vi "Evaluate.vi"(8 "error in (no error)":errorcluster, 10 "Point":dbl[](array[numeric]), 11 "TestObjetive in":refnum<class "TestObjetive.lvclass">) -> (0 "error out":errorcluster, 2 "evaluation":dbl, 3 "TestObjetive out":refnum<class "TestObjetive.lvclass">)   [LabVIEW 2023, in "TestObjetive.lvclass"]
uses:
  TestObjetive.lvclass
  TestObjetive.lvclass/TestObjetive.ctl
  Team_class/OffensivePlay.ctl
  Utilities_class/Utilities.lvclass
panel:
  in  "nearGoal":dbl=1.0 format="%#_13g"
  in  "enemyInSquare":dbl=1.0 format="%#_13g"
  in  "dangerEnemy":dbl=1.0 format="%#_13g"
  in  "factorPass":dbl=1.0 format="%#_13g"
  in  "bestY":dbl=1.0 format="%#_13g"
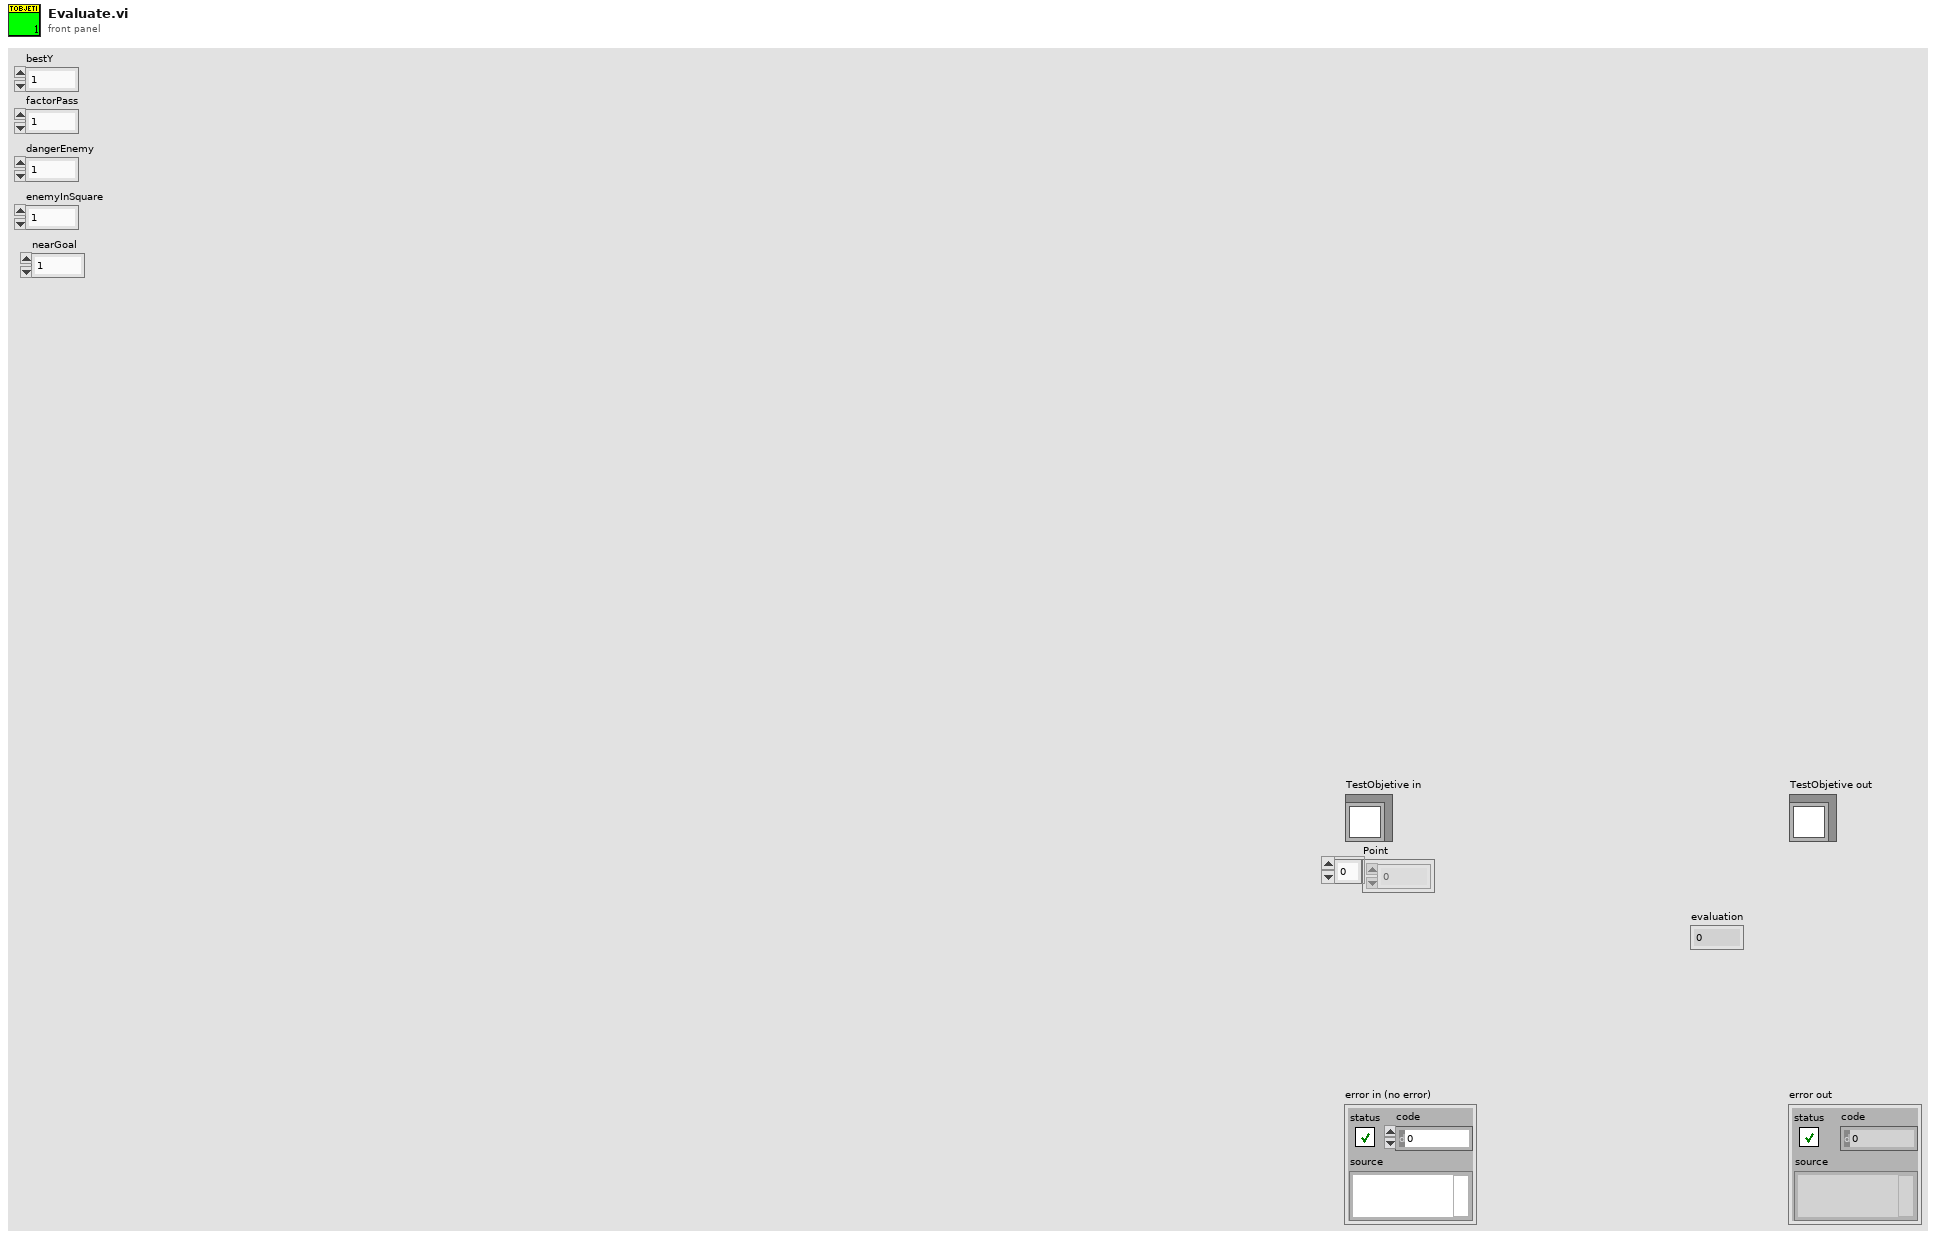
[diagram p1: front panel]
types:
  T1 = typedef "OffensivePlay.ctl" = enum16{"5RobotsPassGamePlay", "5PreparePassGame", "5RobotsKeeperGame", "KeeperPassToStriker", "5RobotsNormalGamePlay", "PrepareKeeperPass", "ACBPass", "ABCPass", "PrepareTriplePass", "TableWithStriker", "TableWith2ndStrikerPlay", "PrepareDoublePass", "PrepareRollToPass", "SimplePass", "PreparePass", "PassToStriker", "BallOutOfField", "PassTo2ndStriker", "StopOffensive", "Prepare Penalty Enemy", "EnemyPossessionAtEnemyField", "EnemyPossesionAtOurField", "TestPlay", "PreparePenaltyAlly", "KickPenaltyAlly", "PrepareKickoffAlly", "PrepareKickoffEnemy", "IndirectEnemy", "DirectEnemy", "PreparePassInGame1", "NormalGame", "DirectKick", "Pass", "Halt", "Timeout", "PassPlay", "PenaltyEnemy"}
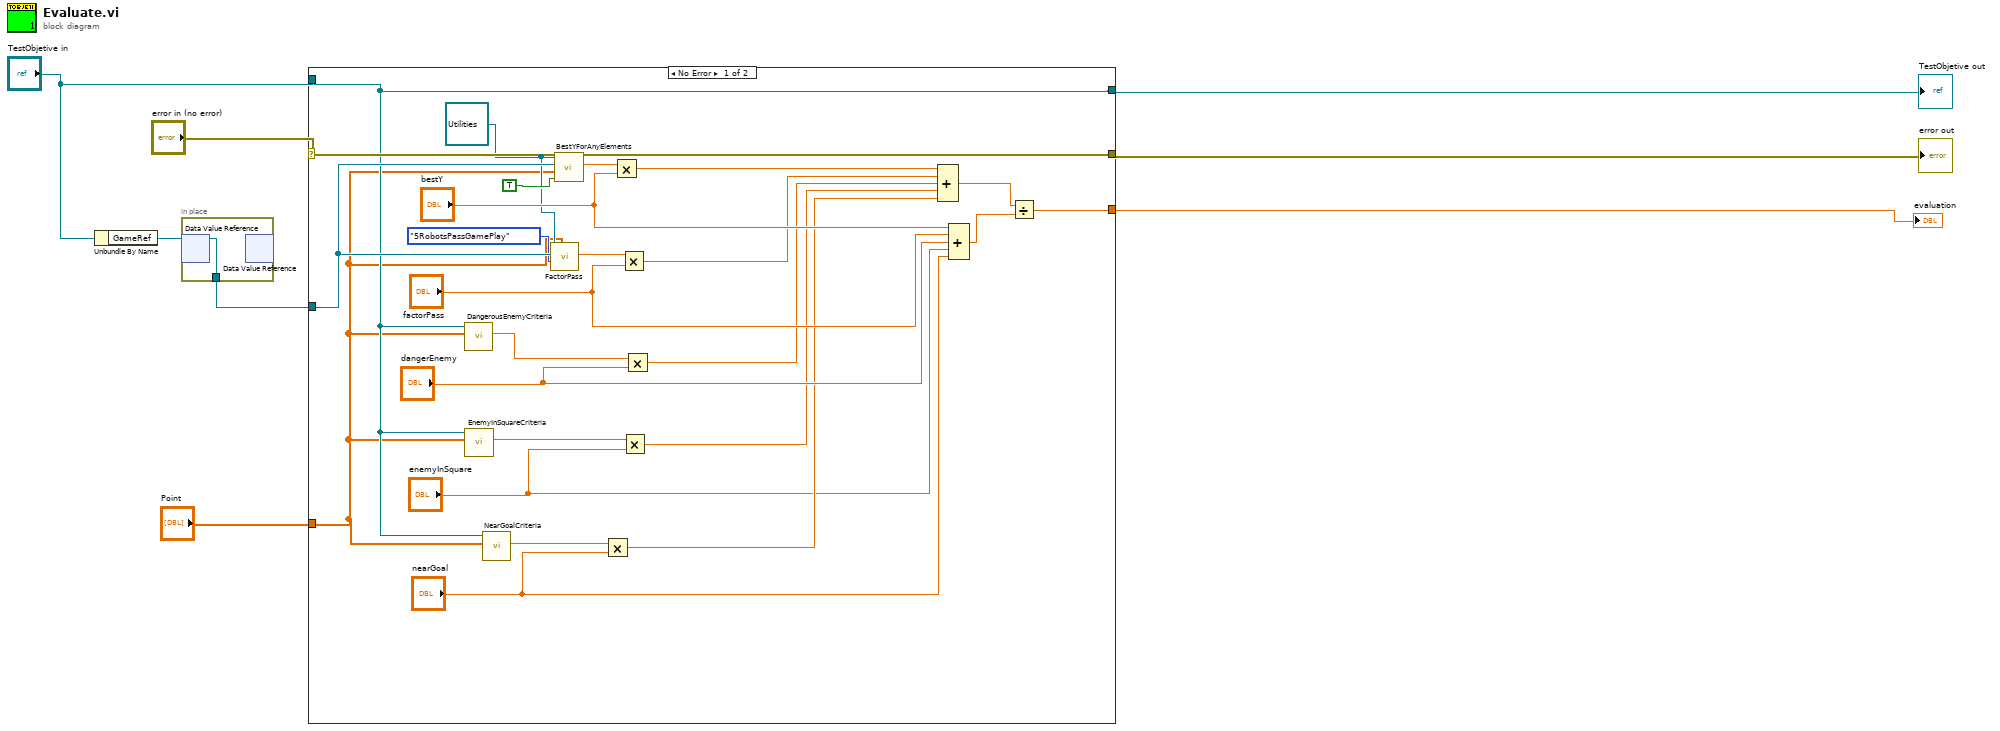
[diagram p0: block diagram]
diagram:
  n1 = Unbundle By Name("TestObjetive in") -> ("GameRef"=w3:refnum<data-value>)
  n2 = in-place {
    in-place-border: [w9] -> w2
    n3 = in-place-dvr #1(w3) -> (w9:refnum<class "Game.lvclass">)  [unwired: 1 out]
    n4 = in-place-dvr #1() -> ()  [unwired: 1 in, 2 out]
  }
  n5 = case shown="No Error" "error in (no error)" {
    selector: "error in (no error)" -> [w34 w36]
    tunnel: [w34 w36] -> w5
    tunnel: "TestObjetive in" -> [w28 w35]
    tunnel: [w28 w35] -> w8
    tunnel: w2 -> [w33 _]
    tunnel: "Point" -> [w10 _]
    tunnel: [w12 _] -> w1
    frame No Error {
      w11 = refnum<class "Utilities.lvclass"> refnum ("Utilities.lvclass")
      n6 = call-dynamic "DangerousEnemyCriteria.vi"("Point"=w10, "TestObjetive in"=w28) -> ("evaluation"=w27:dbl)  [unwired: 7 in, 2 out]
      n7 = call-dynamic "EnemyInSquareCriteria.vi"("Point"=w10, "TestObjetive in"=w28) -> ("evaluation"=w26:dbl)  [unwired: 7 in, 2 out]
      n8 = call-dynamic "NearGoalCriteria.vi"("Point"=w10, "TestObjetive in"=w28) -> ("evaluation"=w25:dbl)  [unwired: 7 in, 2 out]
      n9 = call "FactorPass.vi"("Robot"=w10, "OffensivePlay"=OffensivePlay."5RobotsPassGamePlay", "Game"=w33, "Utilities in"=w11) -> ("Critério de marcação Normalizado"=w31:dbl)  [unwired: 5 in, 2 out]
      n10 = call "BestYForAnyElements.vi"("inimigos"=TRUE, "Position to be analyzed"=w10, "Game"=w33, "Utilities in"=w11) -> ("Goal Gap"=w32:dbl)  [unwired: 6 in, 1 out]
      n11 = Multiply(x=w25, y="nearGoal") -> (x*y=w14:dbl)
      n12 = Multiply(x=w32, y="bestY") -> (x*y=w19:dbl)
      n13 = Multiply(x=w31, y="factorPass") -> (x*y=w17:dbl)
      n14 = Multiply(x=w26, y="enemyInSquare") -> (x*y=w15:dbl)
      n15 = Multiply(x=w27, y="dangerEnemy") -> (x*y=w16:dbl)
      n16 = Compound Arithmetic op=ADD(w19, w17, w16, w15, w14) -> (w18:dbl)
      n17 = Compound Arithmetic op=ADD("bestY", "factorPass", "dangerEnemy", "enemyInSquare", "nearGoal") -> (w20:dbl)
      n18 = Divide(x=w18, y=w20) -> (x/y=w12:dbl)
    }
    frame Error {
    }
  }
  "error out" <- w5
  "TestObjetive out" <- w8
  "evaluation" <- w1
